vi "assignment1.vi"() -> ()   [LabVIEW 2020]
uses:
  <vilib>/Utility/file.llb/Write Delimited Spreadsheet (string).vi
panel:
  out "error out":errorcluster
  in  "delimiter (\\t)":string="\t"
  in  "format (%s)":string="%s"
  in  "stop":bool
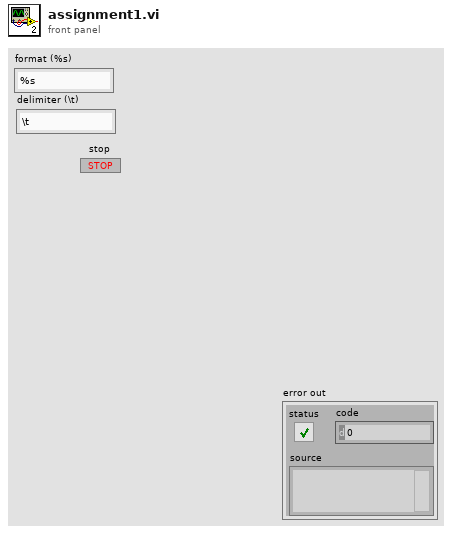
[diagram p1: front panel]
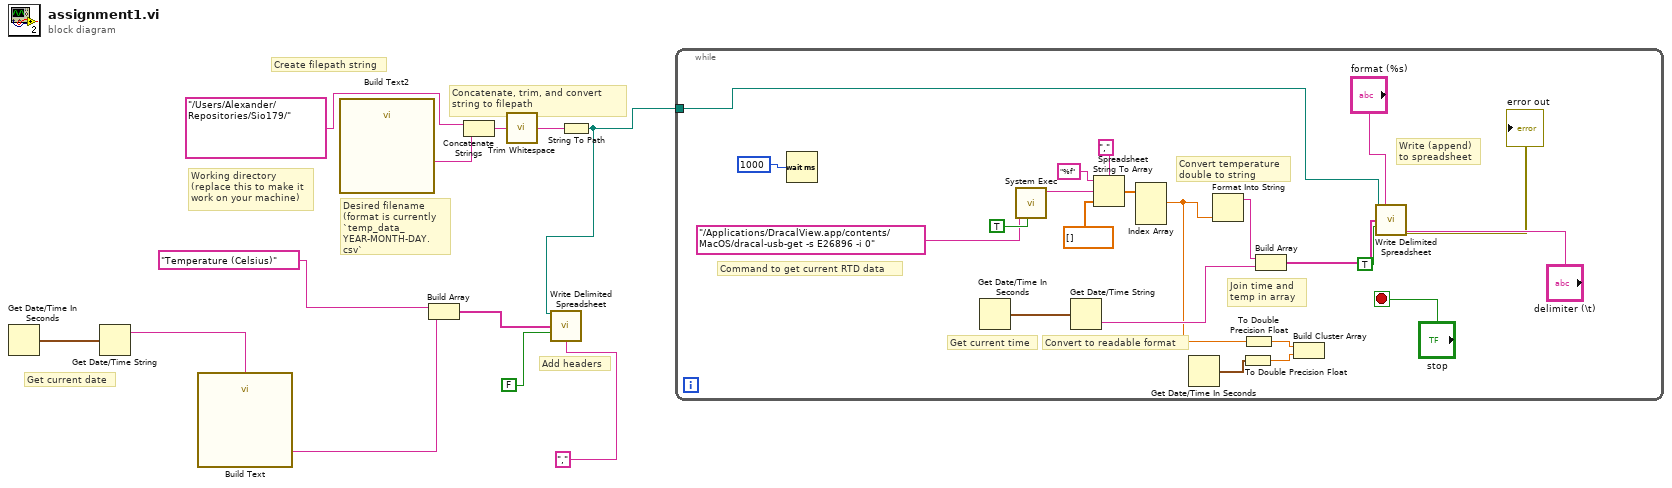
[diagram p0: block diagram]
diagram:
  # "Add headers"
  # "Get current date"
  # "Concatenate, trim, and convert string to filepath"
  # "Desired filename (format is currently `temp_data_YEAR-MONTH-DAY.csv`"
  # "Working directory (replace this to make it work on your machine)"
  # "Create filepath string"
  n1 = Get Date/Time In Seconds() -> (seconds since 1Jan1904=w10:timestamp)
  n2 = Get Date/Time String(seconds (now)=w10) -> (date string=w6:string)  [unwired: 2 in, 1 out]
  n3 = call "Build Text"("date"=w6) -> ("Result"=w9:string)  [unwired: 13 in, 1 out]
  n4 = call "Build Text2"() -> ("Result"=w5:string)  [unwired: 14 in, 1 out]
  n5 = Build Array("Temperature (Celsius)", w9) -> (w8:string[])
  n6 = Concatenate Strings("/Users/Alexander/Repositories/Sio179/", w5) -> (w11:string)
  n7 = call <vilib>:"Trim Whitespace.vi"("string"=w11) -> ("trimmed string"=w12:string)  [unwired: 1 in]
  n8 = String To Path(string=w12) -> (path=w7:path)
  n9 = call-poly <vilib>:"Write Delimited Spreadsheet.vi"("file path (dialog if empty)"=w7, "1D data"=w8, "append to file? (new file:F)"=FALSE, "delimiter (\\t)"=",") -> ()  [unwired: 10 in, 2 out]
  n10 = while {
    tunnel: w7 -> [w17]
    stop <- "stop" stop-if-true
    # "Command to get current RTD data"
    # "Join time and temp in array"
    # "Convert temperature double to string"
    # "Convert to readable format"
    # "Get current time"
    # "Write (append) to spreadsheet"
    n11 = Wait (ms)(milliseconds to wait=u32 1000) -> ()  [unwired: 1 out]
    n12 = Get Date/Time In Seconds() -> (seconds since 1Jan1904=w26:timestamp)
    n13 = call <vilib>:"System Exec.vi"("run minimized? (F)"=TRUE, "command line"="/Applications/DracalView.app/contents/MacOS/dracal-usb-get -s E26896 -i 0") -> ("standard output"=w29:string)  [unwired: 6 in, 3 out]
    n14 = Get Date/Time String(seconds (now)=w26) -> (time string=w27:string)  [unwired: 2 in, 1 out]
    n15 = Spreadsheet String To Array(delimiter (Tab)=",", format string="%f", spreadsheet string=w29, array type (2D Dbl)=dbl[] [] ("Array")) -> (array=w32:dbl[])
    n16 = Index Array(array=w32) -> (element #1=w16:dbl)  [unwired: 3 in, 2 out]
    n17 = Get Date/Time In Seconds() -> (seconds since 1Jan1904=w15:timestamp)
    n18 = Format Into String(w16) -> (resulting string=w18:string)  [unwired: 3 in, 1 out]
    n19 = To Double Precision Float(number=w15) -> (double precision float=w13:dbl)
    n20 = To Double Precision Float(number=w16) -> (double precision float=w14:dbl)
    n21 = Build Array(w18, w27) -> (w19:string[])
    n22 = Build Cluster Array(w14, w13) -> ()  [unwired: 1 out]
    n23 = call-poly <vilib>:"Write Delimited Spreadsheet.vi"("file path (dialog if empty)"=w17, "format (%s)"="format (%s)", "1D data"=w19, "append to file? (new file:F)"=TRUE, "delimiter (\\t)"="delimiter (\\t)") -> ("error out"=→"error out":errorcluster)  [unwired: 9 in, 1 out]
  }
